vi "WriteImageFilePNG.vi"(6 "Use bit depth":bool, 7 "Color Palette":T1[](array[typedef]), 8 "error in":errorcluster, 9 "Image Quality":u32=750, 10 "File Path":path, 11 "Image Reference In":T2) -> (0 "error out":errorcluster, 3 "Image Reference Out":T2)   [LabVIEW 2024, in "OpenLvVision_Image.lvlib" / "File.lvlib"]
doc: "Saves the image to a file in the chosen format."
uses:
  File.lvlib
  Management/TypeDef/Image.ctl
  TypeDef/ColorPaletteValue.ctl
  Management/Management.lvlib
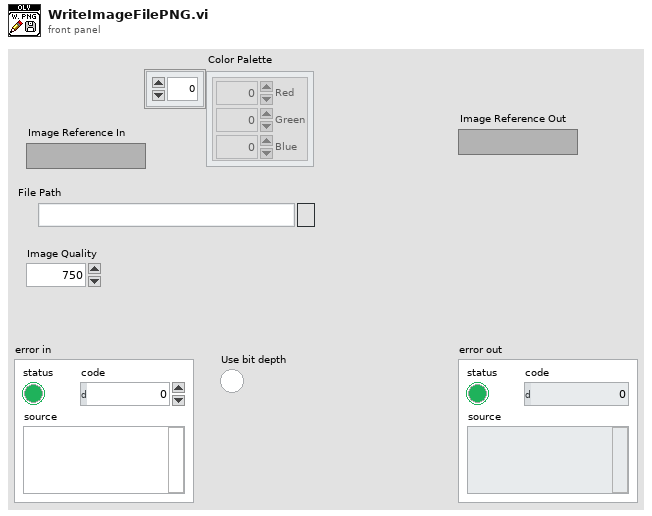
[diagram p1: front panel]
types:
  T1 = typedef "OpenLvVision_Image.lvlib/File.lvlib/ColorPaletteValue.ctl" = cluster{"Red":u8, "Green":u8, "Blue":u8}
  T2 = typedef "OpenLvVision_Image.lvlib/Management.lvlib/Image.ctl" = refnum<image>
  T3 = typedef "IMAQ Image.ctl" = refnum<image>
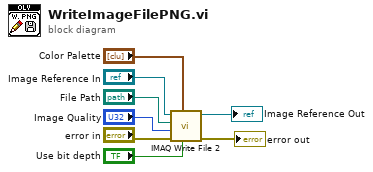
[diagram p0: block diagram]
diagram:
  n1 = call-poly "IMAQ Write File 2"("Use bit depth? (false)"="Use bit depth", "Color Palette"="Color Palette", "error in (no error)"="error in", "Image Quality"="Image Quality", "File Path"="File Path", "Image"="Image Reference In") -> ("error out"=→"error out":errorcluster, "Image Out (duplicate)"=→"Image Reference Out":T3)  [unwired: 4 in]
